vi "[FJC] Calculate Extension.vi"(1 "Temperature (K)":dbl=298.0, 2 "Force (pN)":dbl, 3 "Segment Elasticity (pN/nm)":dbl, 4 "Monomer Length (nm)":dbl, 5 "Contour Length (nm)":dbl, 6 "Segment Length (nm)":dbl) -> (0 "Extension (nm)":dbl)   [LabVIEW 2013]
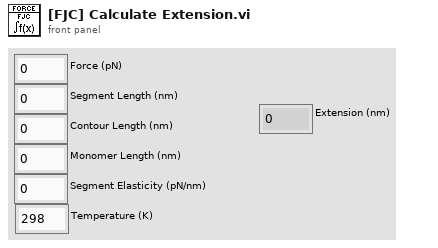
[diagram p1: front panel]
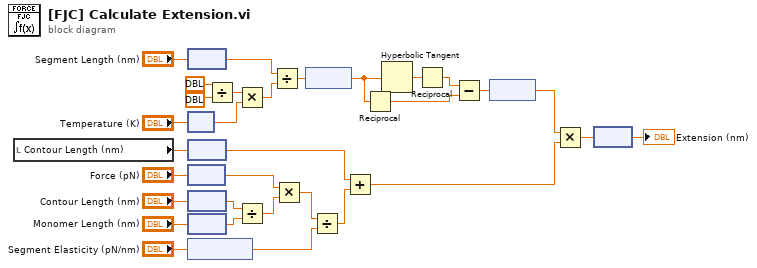
[diagram p0: block diagram]
diagram:
  n1 = local read "Contour Length (nm)"() -> (w24:dbl)
  n2 = node("Segment Length (nm)") -> (w10:dbl[unit])
  n3 = node("Temperature (K)") -> (w17:dbl[unit])
  n4 = node(w24) -> (w18:dbl[unit])
  n5 = node("Force (pN)") -> (w22:dbl[unit])
  n6 = node("Contour Length (nm)") -> (w26:dbl[unit])
  n7 = node("Monomer Length (nm)") -> (w25:dbl[unit])
  n8 = node("Segment Elasticity (pN/nm)") -> (w20:dbl[unit])
  n9 = Divide(x=ext[unit] 8.314472, y=ext[unit] 6.0221415e+23) -> (x/y=w15:ext[unit])
  n10 = Multiply(x=w15, y=w17) -> (x*y=w12:ext[unit])
  n11 = Divide(x=w26, y=w25) -> (x/y=w23:dbl)
  n12 = Divide(x=w10, y=w12) -> (x/y=w9:ext[unit])
  n13 = Multiply(x=w22, y=w23) -> (x*y=w21:dbl[unit])
  n14 = node(w9) -> (w8:ext)
  n15 = Divide(x=w21, y=w20) -> (x/y=w19:dbl[unit])
  n16 = Add(x=w18, y=w19) -> (x+y=w3:dbl[unit])
  n17 = Reciprocal(x=w8) -> (1/x=w6:ext)
  n18 = Hyperbolic Tangent(1:w8) -> (0:w7:ext)
  n19 = Reciprocal(x=w7) -> (1/x=w13:ext)
  n20 = Subtract(x=w13, y=w6) -> (x-y=w5:ext)
  n21 = node(w5) -> (w4:ext[unit])
  n22 = Multiply(x=w4, y=w3) -> (x*y=w2:ext[unit])
  n23 = node(w2) -> (→"Extension (nm)":ext)
